vi "RFH-test-write_readback.vi"() -> ()   [LabVIEW 2020, in "RFH-Reflection_File_Handler.lvlib"]
uses:
  RFH-Reflection_File_Handler.lvlib
  RFH-common_data_format.ctl
panel:
  out "error out":errorcluster
  out "x = y?":T1
  out "Common Format":T2
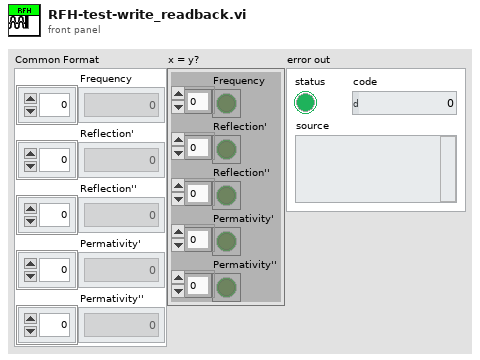
[diagram p1: front panel]
types:
  T1 = cluster{"Frequency":bool[], "Reflection'":bool[], "Reflection''":bool[], "Permativity'":bool[], "Permativity''":bool[]}
  T2 = typedef "RFH-Reflection_File_Handler.lvlib/RFH-common_data_format.ctl" = cluster{"Frequency":dbl[], "Reflection'":dbl[], "Reflection''":dbl[], "Permativity'":dbl[], "Permativity''":dbl[]}
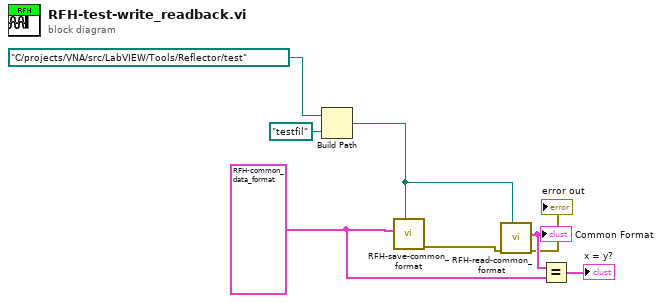
[diagram p0: block diagram]
diagram:
  w3 = T2 {"Frequency"=[200000000.0, 250000000.0, 300000000.0, 350000000.0, 400000000.0, 450000000.0, 500000000.0, 550000000.0, 600000000.0, 650000000.0, 700000000.0, 750000000.0, 800000000.0, 850000000.0, 900000000.0, 950000000.0, 1000000000.0, 1050000000.0, 1100000000.0, 1150000000.0, 1200000000.0, 1250000000.0, 1300000000.0, 1350000000.0, 1400000000.0, 1450000000.0, 1500000000.0, 1550000000.0, 1600000000.0, 1650000000.0, 1700000000.0, 1750000000.0, 1800000000.0, 1850000000.0, 1900000000.0, 1950000000.0, 2000000000.0, 2050000000.0, 2100000000.0, 2150000000.0, 2200000000.0, 2250000000.0, 2300000000.0, 2350000000.0, 2400000000.0, 2450000000.0, 2500000000.0, 2550000000.0, 2600000000.0, 2650000000.0, 2700000000.0, 2750000000.0, 2800000000.0, 2850000000.0, 2900000000.0, 2950000000.0, 3000000000.0, 3050000000.0, 3100000000.0, 3150000000.0, 3200000000.0, 3250000000.0, 3300000000.0, 3350000000.0, 3400000000.0, 3450000000.0, 3500000000.0, 3550000000.0, 3600000000.0, 3650000000.0, 3700000000.0, 3750000000.0, 3800000000.0, 3850000000.0, 3900000000.0, 3950000000.0, 4000000000.0, 4050000000.0, 4100000000.0, 4150000000.0, 4200000000.0, 4250000000.0, 4300000000.0, 4350000000.0, 4400000000.0, 4450000000.0, 4500000000.0, 4550000000.0, 4600000000.0, 4650000000.0, 4700000000.0, 4750000000.0, 4800000000.0, 4850000000.0, 4900000000.0, 4950000000.0, 5000000000.0, 5050000000.0, 5100000000.0, 5150000000.0, 5200000000.0, 5250000000.0, 5300000000.0, 5350000000.0, 5400000000.0, 5450000000.0, 5500000000.0, 5550000000.0, 5600000000.0, 5650000000.0, 5700000000.0, 5750000000.0, 5800000000.0, 5850000000.0, 5900000000.0, 5950000000.0, 6000000000.0, 6050000000.0, 6100000000.0, 6150000000.0, 6200000000.0, 6250000000.0, 6300000000.0, 6350000000.0, 6400000000.0, 6450000000.0, 6500000000.0, 6550000000.0, 6600000000.0, 6650000000.0, 6700000000.0, 6750000000.0, 6800000000.0, 6850000000.0, 6900000000.0, 6950000000.0, 7000000000.0, 7050000000.0, 7100000000.0, 7150000000.0, 7200000000.0, 7250000000.0, 7300000000.0, 7350000000.0, 7400000000.0, 7450000000.0, 7500000000.0, 7550000000.0, 7600000000.0, 7650000000.0, 7700000000.0, 7750000000.0, 7800000000.0, 7850000000.0, 7900000000.0, 7950000000.0, 8000000000.0, 8050000000.0, 8100000000.0, 8150000000.0, 8200000000.0, 8250000000.0, 8300000000.0, 8350000000.0, 8400000000.0, 8450000000.0, 8500000000.0], "Reflection'"=[0.9811679999999999, 0.9704271666666666, 0.9577146666666666, 0.9428123333333334, 0.9261786666666668, 0.907561, 0.8870205000000001, 0.8649226666666667, 0.8414076666666667, 0.8161839999999999, 0.7901213333333331, 0.7626563333333333, 0.734536, 0.7053663333333334, 0.6757843333333332, 0.6449838333333333, 0.6142455, 0.5831633333333333, 0.5518835, 0.5199753333333333, 0.4891546666666666, 0.4588021666666666, 0.4275428333333333, 0.3969135, 0.364168, 0.3330248333333333, 0.30421650000000006, 0.27603300000000003, 0.24708549999999999, 0.21858966666666668, 0.19152466666666668, 0.16355566666666665, 0.13698649999999998, 0.11144866666666665, 0.08612061666666666, 0.06127085000000001, 0.037459933333333334, 0.013727133333333334, -0.009271640000000001, -0.030811866666666663, -0.05203318333333334, -0.07206038333333334, -0.09145788333333334, -0.110938, -0.13037983333333333, -0.14924099999999998, -0.1672515, -0.18404533333333337, -0.20024616666666664, -0.2155878333333333, -0.230168, -0.24511433333333332, -0.25995433333333334, -0.27423616666666667, -0.28797616666666664, -0.3009266666666666, -0.3130288333333333, -0.3252296666666667, -0.3368058333333333, -0.34827616666666666, -0.359211, -0.36978633333333333, -0.37993666666666664, -0.39007833333333336, -0.3996283333333333, -0.40843366666666664, -0.41708266666666666, -0.42569049999999997, -0.4339691666666667, -0.4419376666666666, -0.44993666666666665, -0.4577161666666667, -0.4650386666666666, -0.4720925, -0.4787776666666666, -0.48498816666666666, -0.491353, -0.49758949999999996, -0.503572, -0.5095063333333334, -0.515308, -0.5208091666666665, -0.5257583333333334, -0.5304418333333333, -0.5353713333333333, -0.5396241666666667, -0.5444371666666666, -0.5492151666666666, -0.5537789999999999, -0.5582793333333333, -0.5623035000000001, -0.5661833333333334, -0.5714568333333333, -0.5751411666666667, -0.5764433333333333, -0.5820106666666667, -0.5843811666666667, -0.5884786666666666, -0.591206, -0.5945571666666667, -0.5965643333333334, -0.5990993333333333, -0.6037241666666667, -0.6045403333333333, -0.6085461666666666, -0.6095265000000001, -0.6134408333333333, -0.6154253333333334, -0.618072, -0.6188738333333333, -0.622963, -0.6244808333333334, -0.627542, -0.6307856666666668, -0.6296811666666666, -0.6322396666666666, -0.6336463333333333, -0.6351378333333333, -0.6369575, -0.6383753333333333, -0.6385998333333334, -0.640986, -0.6437931666666667, -0.644945, -0.6471665, -0.647281, -0.6483070000000001, -0.648991, -0.6500423333333333, -0.6508966666666666, -0.6534143333333333, -0.6556886666666667, -0.6528055, -0.6543816666666668, -0.655597, -0.6592961666666667, -0.6591741666666666, -0.6584746666666667, -0.660096, -0.6603943333333333, -0.6602706666666666, -0.66237, -0.6635966666666667, -0.664228, -0.6664863333333333, -0.6642278333333332, -0.6677956666666667, -0.663748, -0.6656083333333334, -0.6656823333333334, -0.6679396666666667, -0.6694458333333334, -0.669457, -0.6700533333333333, -0.668859, -0.6717126666666666, -0.6699758333333333, -0.6722976666666667, -0.6698666666666666, -0.6701638333333334, -0.6707603333333333, -0.6723083333333334, -0.6727203333333334, -0.6715008333333333, -0.6731885000000001, -0.6722051666666666, -0.6709063333333334], "Reflection''"=[-0.18390266666666666, -0.2286161666666667, -0.2726028333333333, -0.315554, -0.35731033333333334, -0.3978873333333333, -0.43700883333333335, -0.4743386666666667, -0.5107853333333333, -0.5451795, -0.5779658333333334, -0.6089296666666667, -0.6383236666666666, -0.6657941666666667, -0.6924481666666665, -0.7157701666666667, -0.7380271666666666, -0.7586628333333333, -0.7772289999999998, -0.7943313333333332, -0.8091103333333334, -0.8239088333333333, -0.8370093333333334, -0.8489666666666666, -0.8594368333333332, -0.8662163333333334, -0.8721021666666666, -0.8782461666666666, -0.8838926666666667, -0.8872695, -0.890682, -0.8928505000000001, -0.8932118333333334, -0.8936696666666665, -0.8933531666666666, -0.8916791666666667, -0.8897285, -0.8870054999999999, -0.8834439999999999, -0.8794825000000001, -0.8752681666666667, -0.8706665, -0.8656218333333333, -0.8611851666666666, -0.8560095, -0.8500366666666667, -0.8434998333333333, -0.8362155000000001, -0.8290581666666667, -0.8224531666666667, -0.816468, -0.8098605, -0.8026413333333334, -0.7953786666666667, -0.788012, -0.7805653333333332, -0.7731794999999999, -0.7654048333333333, -0.7573175, -0.7498346666666666, -0.7421165, -0.734417, -0.726916, -0.7196141666666668, -0.7122935, -0.7049883333333332, -0.6977261666666666, -0.6900513333333335, -0.682371, -0.6748215000000001, -0.6674859999999999, -0.6604015, -0.6533501666666667, -0.6463016666666667, -0.639533, -0.6326256666666666, -0.6261439999999999, -0.6185316666666666, -0.6114413333333333, -0.6044828333333334, -0.5980478333333333, -0.5918246666666667, -0.5853621666666666, -0.5789961666666668, -0.5726873333333333, -0.5665745000000001, -0.5599855, -0.5534091666666666, -0.5470866666666667, -0.5411163333333334, -0.5355166666666668, -0.5302743333333334, -0.5238203333333332, -0.5178346666666667, -0.5113105, -0.5053181666666667, -0.5009641666666667, -0.4960235, -0.4898275, -0.4832906666666667, -0.47789483333333327, -0.47353616666666665, -0.46685683333333333, -0.46429349999999997, -0.4610175, -0.452423, -0.4478393333333333, -0.4434646666666667, -0.437527, -0.4326468333333333, -0.4288546666666666, -0.42489683333333333, -0.4197688333333333, -0.41405866666666674, -0.4112111666666666, -0.40688466666666673, -0.400625, -0.3971343333333333, -0.39237883333333334, -0.387978, -0.3835685, -0.37902016666666666, -0.37182733333333334, -0.370782, -0.36673416666666664, -0.3632761666666667, -0.3606463333333334, -0.35705933333333334, -0.3523928333333333, -0.34868683333333333, -0.3453158333333333, -0.34010650000000003, -0.335059, -0.3334671666666667, -0.32942466666666664, -0.3279176666666666, -0.32324833333333336, -0.3217601666666667, -0.3166926666666667, -0.31151799999999996, -0.30896166666666663, -0.3069305, -0.30250066666666664, -0.3002848333333333, -0.2952815, -0.29362816666666663, -0.2897551666666667, -0.2865911666666667, -0.28160883333333336, -0.27978016666666666, -0.27671566666666664, -0.273685, -0.27090216666666667, -0.26874216666666667, -0.2684493333333333, -0.26515816666666664, -0.2554476666666667, -0.255299, -0.255309, -0.25261750000000005, -0.24982400000000002, -0.24829933333333332, -0.244942, -0.24258316666666666, -0.24083433333333334, -0.23801850000000002, -0.23438983333333333], "Permativity'"=[78.93663333333332, 78.94888333333334, 78.96293333333334, 78.97188333333334, 78.97983333333333, 78.98018333333333, 78.97875, 78.97795, 78.97448333333334, 78.97016666666666, 78.95673333333333, 78.93041666666666, 78.89976666666666, 78.87676666666667, 78.8567, 78.83678333333334, 78.82235, 78.80666666666667, 78.78806666666667, 78.76733333333333, 78.74664999999999, 78.72316666666667, 78.69788333333334, 78.67464999999999, 78.64558333333333, 78.61561666666667, 78.58396666666665, 78.55160000000001, 78.52289999999999, 78.49946666666666, 78.47266666666667, 78.4432, 78.40578333333333, 78.36273333333334, 78.31556666666667, 78.26248333333335, 78.21811666666666, 78.18168333333332, 78.14883333333333, 78.11918333333334, 78.07478333333334, 78.01858333333332, 77.9623, 77.9089, 77.85308333333333, 77.79565000000001, 77.74053333333335, 77.67988333333334, 77.61906666666667, 77.55818333333333, 77.49573333333335, 77.43308333333333, 77.37259999999999, 77.31125, 77.24626666666667, 77.18149999999999, 77.1134, 77.04303333333334, 76.97598333333333, 76.91096666666667, 76.84493333333334, 76.77701666666667, 76.70603333333334, 76.63163333333334, 76.55348333333333, 76.473, 76.39448333333333, 76.31466666666667, 76.23389999999999, 76.1549, 76.07331666666668, 75.99543333333334, 75.92129999999999, 75.84635, 75.77014999999999, 75.68916666666667, 75.60459999999999, 75.52648333333332, 75.44151666666667, 75.34126666666666, 75.25513333333332, 75.15766666666667, 75.06868333333334, 74.98223333333333, 74.90353333333333, 74.82118333333332, 74.73935, 74.67506666666667, 74.58818333333333, 74.51265000000001, 74.44328333333334, 74.38320000000002, 74.31563333333334, 74.24968333333334, 74.16988333333332, 74.09578333333333, 74.00636666666666, 73.91853333333334, 73.8309, 73.70985, 73.60191666666667, 73.50743333333334, 73.41134999999998, 73.32168333333333, 73.23235, 73.13718333333333, 73.05796666666667, 73.00021666666667, 72.90455, 72.80676666666666, 72.70976666666667, 72.5964, 72.49708333333332, 72.40601666666667, 72.31665, 72.2265, 72.14274999999999, 72.03043333333333, 71.8957, 71.78861666666666, 71.69296666666666, 71.58738333333334, 71.45353333333334, 71.34521666666666, 71.22840000000001, 71.11028333333333, 70.99038333333333, 70.88350000000001, 70.7545, 70.61041666666667, 70.45033333333333, 70.32138333333334, 70.15016666666666, 70.02268333333335, 69.89023333333333, 69.78101666666667, 69.69281666666667, 69.59545000000001, 69.46701666666667, 69.32775, 69.20866666666667, 69.09708333333333, 68.98383333333334, 68.84043333333334, 68.719, 68.62248333333334, 68.52901666666666, 68.40668333333333, 68.28425, 68.1804, 68.06385, 67.9234, 67.78888333333335, 67.67813333333335, 67.54055000000001, 67.39300000000001, 67.2665, 67.11851666666668, 66.94045, 66.77829999999999, 66.58421666666668, 66.40941666666667, 66.20936666666667, 66.06416666666667, 65.90758333333333, 65.77865, 65.65801666666667], "Permativity''"=[0.7556815, 1.1030066666666667, 1.324825, 1.519065, 1.695285, 1.869565, 2.0301633333333333, 2.2037400000000003, 2.3843666666666663, 2.586755, 2.8098533333333333, 3.0277483333333333, 3.2289500000000007, 3.4230583333333335, 3.6212983333333337, 3.814125, 4.009546666666666, 4.211425, 4.410323333333333, 4.607175000000001, 4.80863, 5.009618333333333, 5.209135000000001, 5.4083716666666675, 5.607124999999999, 5.802503333333334, 5.996446666666667, 6.1868050000000006, 6.372369999999999, 6.560138333333334, 6.7580550000000015, 6.95972, 7.164176666666666, 7.367303333333333, 7.5638016666666665, 7.75191, 7.93702, 8.126181666666666, 8.319411666666666, 8.520785000000002, 8.728531666666667, 8.933146666666667, 9.131995000000002, 9.330473333333334, 9.524988333333333, 9.714843333333333, 9.904376666666666, 10.090566666666666, 10.271533333333332, 10.453633333333334, 10.640316666666665, 10.828533333333334, 11.018933333333331, 11.211916666666667, 11.404499999999999, 11.594366666666668, 11.780783333333332, 11.962666666666665, 12.142666666666665, 12.325466666666665, 12.514216666666664, 12.704300000000003, 12.899000000000001, 13.089816666666666, 13.273933333333332, 13.449933333333334, 13.623316666666668, 13.796149999999999, 13.969483333333335, 14.143033333333335, 14.318283333333332, 14.495750000000001, 14.671999999999999, 14.847216666666668, 15.018083333333335, 15.188183333333333, 15.356216666666667, 15.524033333333335, 15.694716666666666, 15.876850000000003, 16.046583333333334, 16.2101, 16.368666666666666, 16.539283333333334, 16.7144, 16.88553333333333, 17.04478333333333, 17.20563333333333, 17.355249999999998, 17.49846666666667, 17.685066666666668, 17.85195, 18.013333333333332, 18.17653333333333, 18.337966666666667, 18.479083333333335, 18.625116666666667, 18.779766666666667, 18.943116666666665, 19.107000000000003, 19.268816666666666, 19.444733333333332, 19.59896666666667, 19.74866666666667, 19.893366666666665, 20.039450000000002, 20.17935, 20.33545, 20.46545, 20.60826666666667, 20.752333333333333, 20.897000000000002, 21.0534, 21.2346, 21.417683333333333, 21.589883333333333, 21.76765, 21.9657, 22.115049999999997, 22.270233333333334, 22.42396666666667, 22.582783333333335, 22.731583333333333, 22.89446666666667, 23.056266666666662, 23.182683333333333, 23.291700000000002, 23.41588333333333, 23.535283333333336, 23.6668, 23.799116666666666, 23.9341, 24.074583333333333, 24.21745, 24.340899999999994, 24.462100000000003, 24.58543333333333, 24.72243333333333, 24.835449999999998, 24.95923333333333, 25.09775, 25.30546666666667, 25.44231666666667, 25.567916666666665, 25.697316666666666, 25.83315, 25.976183333333335, 26.142033333333334, 26.280250000000006, 26.406566666666667, 26.528816666666668, 26.682516666666668, 26.796483333333338, 26.921066666666665, 27.021266666666666, 27.091183333333333, 27.146866666666668, 27.222050000000007, 27.30946666666667, 27.4169, 27.52916666666667, 27.643699999999995, 27.769933333333338, 27.87315, 27.9697, 28.078233333333333, 28.18771666666667]} ("Common Format 3")
  n1 = Build Path(base path=path "C:/projects/VNA/src/LabVIEW/Tools/Reflector/test", name or relative path=path "testfil") -> (appended path=w5:path)
  n2 = call "RFH-save-common_format.vi"("file path (use dialog)"=w5, "Common Format"=w3) -> ("error out"=w6:errorcluster)  [unwired: 9 in]
  n3 = call "RFH-read-common_format.vi"("file path (dialog if empty)"=w5, "error in"=w6) -> ("error out"=→"error out":errorcluster, "Common Format"=w4:T2)  [unwired: 8 in]
  "Common Format" <- w4
  n4 = Equal?(x=w4, y=w3) -> (x = y?=→"x = y?":T1)
